vi "Counter.vi"(7 "Set (f)":bool, 8 "error in (no error)":errorcluster, 11 "Counter In":i32) -> (0 "error out":errorcluster, 3 "Counter Out":i32)   [LabVIEW 2018, in "ScopePlugins.lvlib"]
uses:
  ScopePlugins.lvlib
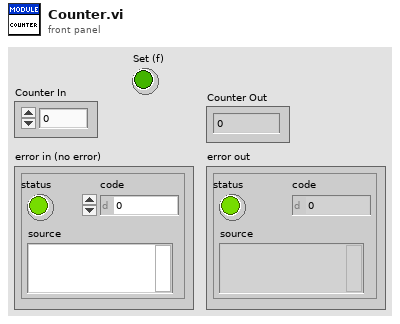
[diagram p1: front panel]
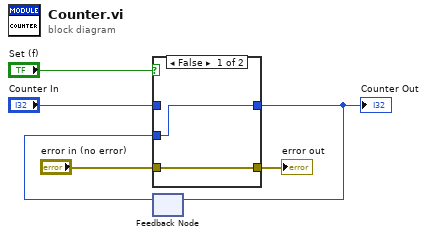
[diagram p0: block diagram]
diagram:
  n1 = feedback #1() -> (w1:i32)  [unwired: 1 in]
  n2 = case shown="False" "Set (f)" {
    tunnel: "Counter In" -> [_ w10]
    tunnel: [w7 w10] -> w2
    tunnel: "error in (no error)" -> [w8 w9]
    tunnel: [w8 w9] -> w3
    tunnel: w1 -> [w7 _]
    frame False {
    }
    frame True {
    }
  }
  "error out" <- w3
  "Counter Out" <- w2
  n3 = feedback-in #1(w2) -> ()
